vi "FNL.vi"(0 "System no.":i32=1 min=1 max=4 step=1, 2 "Affected axes":string[](array[string]), 3 "All axes?":bool, 4 "Axis identifier?":bool=TRUE, 5 "error in":errorcluster) -> (19 "error out":errorcluster)   [LabVIEW 2020]
doc: "This VI starts a fast move to negative limit of the specified axes.Use #7 polling to determine end of this referencing procedure.\n\nC-843, C-843.PM: If All axes? = TRUE, then Axis identifier? must be TRUE\n\nC-867, C-884: If not, you can use FRF instead and set parameter no. 0x70 to select which sensor is to use for referencing. See controller user manual for details. \n\nE-755: If All axes? = TRUE, then Axis identifier? can be FALSE. Command not available for E-755.101\n\nC-867, C-877, C-884, E-871, E-873, E-874, Hydra, Pollux, Mercury_GCS: If All axes? = TRUE, then Axis identifier? must be TRUE. Servo must be enabled with SVO for the commanded axis prior to using this command (closed-loop operation).\nThe reference mode must be set to \"1\" (factory default) with the RON command if referencing is to be done by performing a reference move. \nThe negative limit switch of the mechanics is used to determine the negative physical limit of the travel range. The difference of VALUE_AT_REF_POS (parameter ID 0x16) and DISTANCE_REF_TO_N_LIM (parameter ID 0x17) is set as the current position when the axis is at the negative limit switch (value can be negative). If the soft limits (MAX_TRAVEL_RANGE_POS, parameter ID 0x15, and MAX_TRAVEL_RANGE_NEG, parameter ID 0x30) are used to reduce the travel range, the limit switches can not be used for reference moves. FNL and FPL commands will provoke an error message, and only the reference switch can be used for a reference move (FRF command). See user manual for details and specifics. \n\nE-861: If All axes? = TRUE, then Axis identifier? must be TRUE. The reference mode must be set to \"1\" (factory default) with the RON command if referencing is to be done by performing a reference move. \nThe negative limit switch of the mechanics is used to determine the negative physical limit of the travel range. The difference of VALUE_AT_REF_POS (parameter ID 0x16) and DISTANCE_REF_TO_N_LIM (parameter ID 0x17) is set as the current position when the axis is at the negative limit switch (value can be negative). If the soft limits (MAX_TRAVEL_RANGE_POS, parameter ID 0x15, and MAX_TRAVEL_RANGE_NEG, parameter ID 0x30) are used to reduce the travel range, the limit switches can not be used for reference moves. FNL and FPL commands will provoke an error message, and only the reference switch can be used for a reference move (FRF command)."
panel:
  # "This vi starts a fast move to negative limit of the specified axes.\nUse #7 polling to determine end of this referencing procedure."
  # "If all axes: use"
  # "FNL"
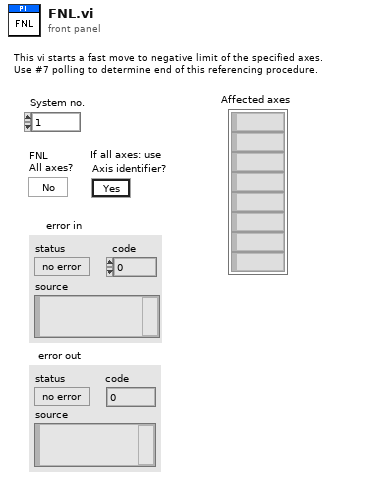
[diagram p1: front panel]
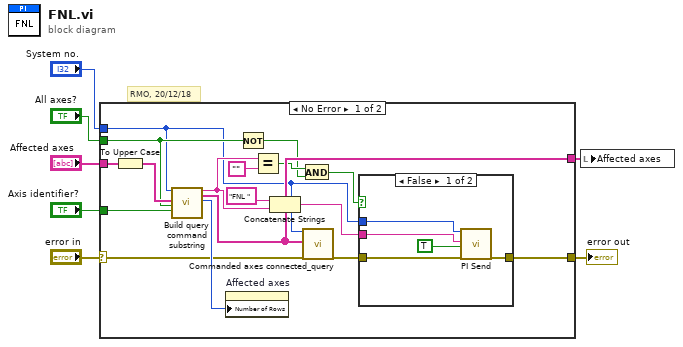
[diagram p0: block diagram]
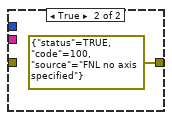
[diagram p2: hidden frame]
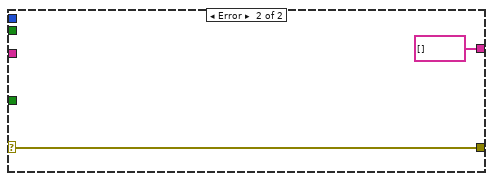
[diagram p3: hidden frame]
diagram:
  # "RMO, 20/12/18"
  n1 = case shown="No Error" "error in" {
    selector: "error in" -> [w8 w31]
    tunnel: "Affected axes" -> [w23 _]
    tunnel: [w20 w31] -> w6
    tunnel: "Axis identifier?" -> [w18 _]
    tunnel: "System no." -> [w9 _]
    tunnel: [w15 string[] [] ("Axes to query out")] -> w3
    tunnel: "All axes?" -> [w14 _]
    frame No Error {
      n2 = To Upper Case(1:w23) -> (0:w19:string[])
      n3 = call "Build query command substring.vi"("System no."=w9, "Axes to query in"=w19, "Query\nAll axes?"=w14, "For all axes: use\nAxis identifier?"=w18) -> ("Command substring"=w17:string, "Axes to query out"=w15:string[], "Number of rows"=w16:u32)  [unwired: 2 in, 11 out]
      n4 = property on="Affected axes" class="Arr (strict)"("Number of Rows"=w16) -> ()  [unwired: 2 in, 2 out]
      n5 = Not(x=w14) -> (.not. x?=w12:bool)
      n6 = Equal?(x=w17, y="" ("x")) -> (x = y?=w13:bool)
      n7 = Concatenate Strings("FNL ", w17) -> (w10:string)
      n8 = And(x=w13, y=w12) -> (x .and. y?=w21:bool)
      n9 = call "Commanded axes connected_query.vi"("System no."=w9, "Commanded axes"=w15, "error in"=w8) -> ("error out"=w11:errorcluster)  [unwired: 1 in, 15 out]
      n10 = case shown="False" w21 {
        tunnel: [w28 errorcluster {"status"=TRUE, "code"=100, "source"="FNL no axis specified"} ("error out")] -> w20
        tunnel: w11 -> [w29 _]
        tunnel: w10 -> [w26 _]
        tunnel: w9 -> [w25 _]
        frame False {
          n11 = call "PI Send.vi"("System no."=w25, "String to send"=w26, "Attach termination char.?"=TRUE ("Attach Linefeed?"), "error in"=w29) -> ("error out"=w28:errorcluster)  [unwired: 2 in, 13 out]
        }
        frame True {
        }
      }
    }
    frame Error {
    }
  }
  "error out" <- w6
  n12 = local write "Affected axes"(w3) -> ()
